vi "RunTest2.vi"(8 "error in (no error)":errorcluster, 11 "Prueba05 in":refnum<class "Prueba05.lvclass">) -> (0 "error out":errorcluster, 2 "resultado":string, 3 "Prueba05 out":refnum<class "Prueba05.lvclass">)   [LabVIEW 2019]
uses:
  Prueba/Prueba.lvclass
  Prueba05.lvclass
  <vilib>/Utility/miscctls.llb/LVRowAndColumnTypeDef.ctl
  Prueba04/Control/Slide.ctl
  Prueba04/Prueba04.lvclass
  QMH/User Event - Stop/User Event - Stop.lvlib
  QMH/Message Queue/Message Queue.lvlib
  <vilib>/Utility/error.llb/Error Cluster From Error Code.vi
  <vilib>/ErrorRing/Error Ring.xnode
  QMH/Message Queue/Enqueue Message (Single).vi
  ClusterGEN.ctl
  <vilib>/Utility/error.llb/DialogType.ctl
  D:/REPO/GitHub/procal/Pruebas/Prueba/Prueba.lvclass
panel:
  out "cumple_no_cumple":bool
  in  "Tab":enum32{"Page 1", "Page 2"}(tab)
  in  "generar_1":bool
  out "frecuencia":dbl
  in  "seguir":bool
  out "voltaje1":dbl format="%.1f"
  out "frecuencia1":dbl format="%.1f"
  in  "AjusteAmp":T1=50.0 caption="Ajuste de amplitud [mV]" scale=0.0..500.0
  in  "guardar":bool
  in  "Tabla_A":string[][](table)
  out "voltaje2":dbl format="%.1f"
  out "frecuencia2":dbl format="%.1f"
  out "no_cumple":bool
  out "cumple":bool
  out "voltaje2":dbl format="%.1f"
  in  "generar_2":bool
  out "frecuencia2":dbl
  in  "salir":bool
  # "Generación Señal de Prueba"
  # "Hz"
  # "Frecuencia"
  # "5. Ponderaciones frecuenciales y temporales a 1 KHz. IEC 61672-3: 2006 Cláusula 13"
  # "Monitoreo"
  # "Frecuencia"
  # "Hz"
  # "Voltaje"
  # "mV"
  # "Hz"
  # "mV"
  # "Cumple"
  # "No Cumple"
  # "Monitoreo"
  # "Frecuencia"
  # "Hz"
  # "Voltaje"
  # "mV"
  # "Voltaje"
  # "Frecuencia"
  # "5. Ponderaciones frecuenciales y temporales a 1 KHz. IEC 61672-3: 2006 Cláusula 13"
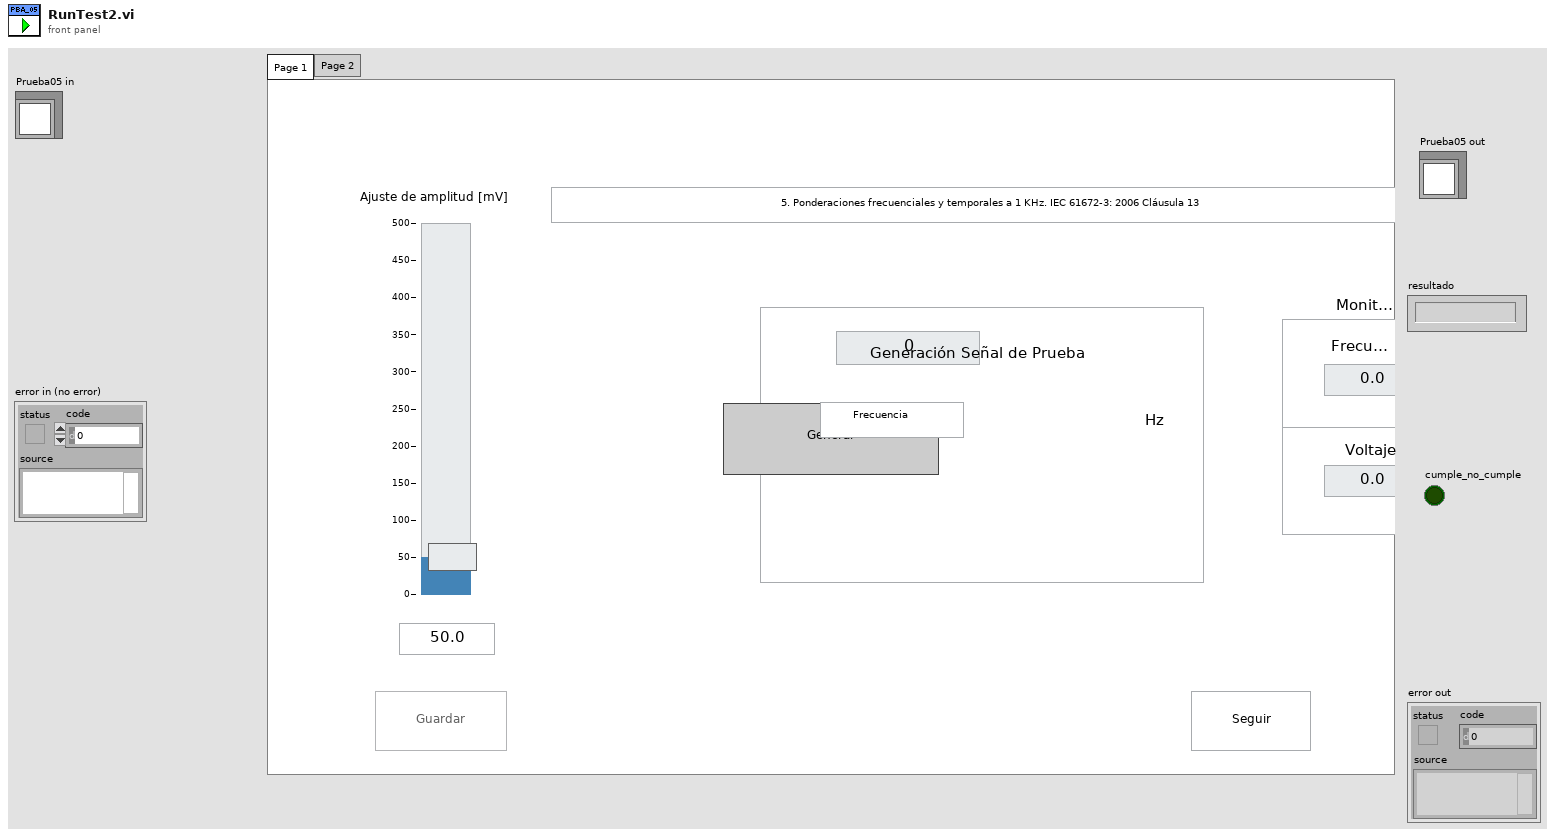
[diagram p1: front panel]
types:
  T1 = typedef "Prueba04.lvclass/Slide.ctl" = dbl
  T2 = typedef "Message Queue.lvlib/All Message Queues.ctl" = cluster{"MHL":refnum<queue>, "Inst_CNT90":refnum<queue>, "Inst_DS360":refnum<queue>, "Inst_Keithley2002":refnum<queue>, "Inst_DAQ":refnum<queue>, "BD":refnum<queue>, "Pistofono":refnum<queue>, "Nexus":refnum<queue>}
  T3 = enum8{"Enabled", "Disabled", "Disabled and Grayed Out"}
  T4 = typedef "LVRowAndColumnTypeDef.ctl" = cluster{"Row":i32, "Column":i32}
  T5 = enum32{"Page 1", "Page 2", "Page 3", "Page 4", "Page 5", "Page 6", "Page 7"}
  T6 = typedef "Prueba05.lvclass/ClusterGEN.ctl" = cluster{"frec":dbl, "amp":dbl}
  T7 = cluster{"ControlName":string, "ControlReference":refnum<vi>}[]
  T8 = typedef "DialogType.ctl" = u16
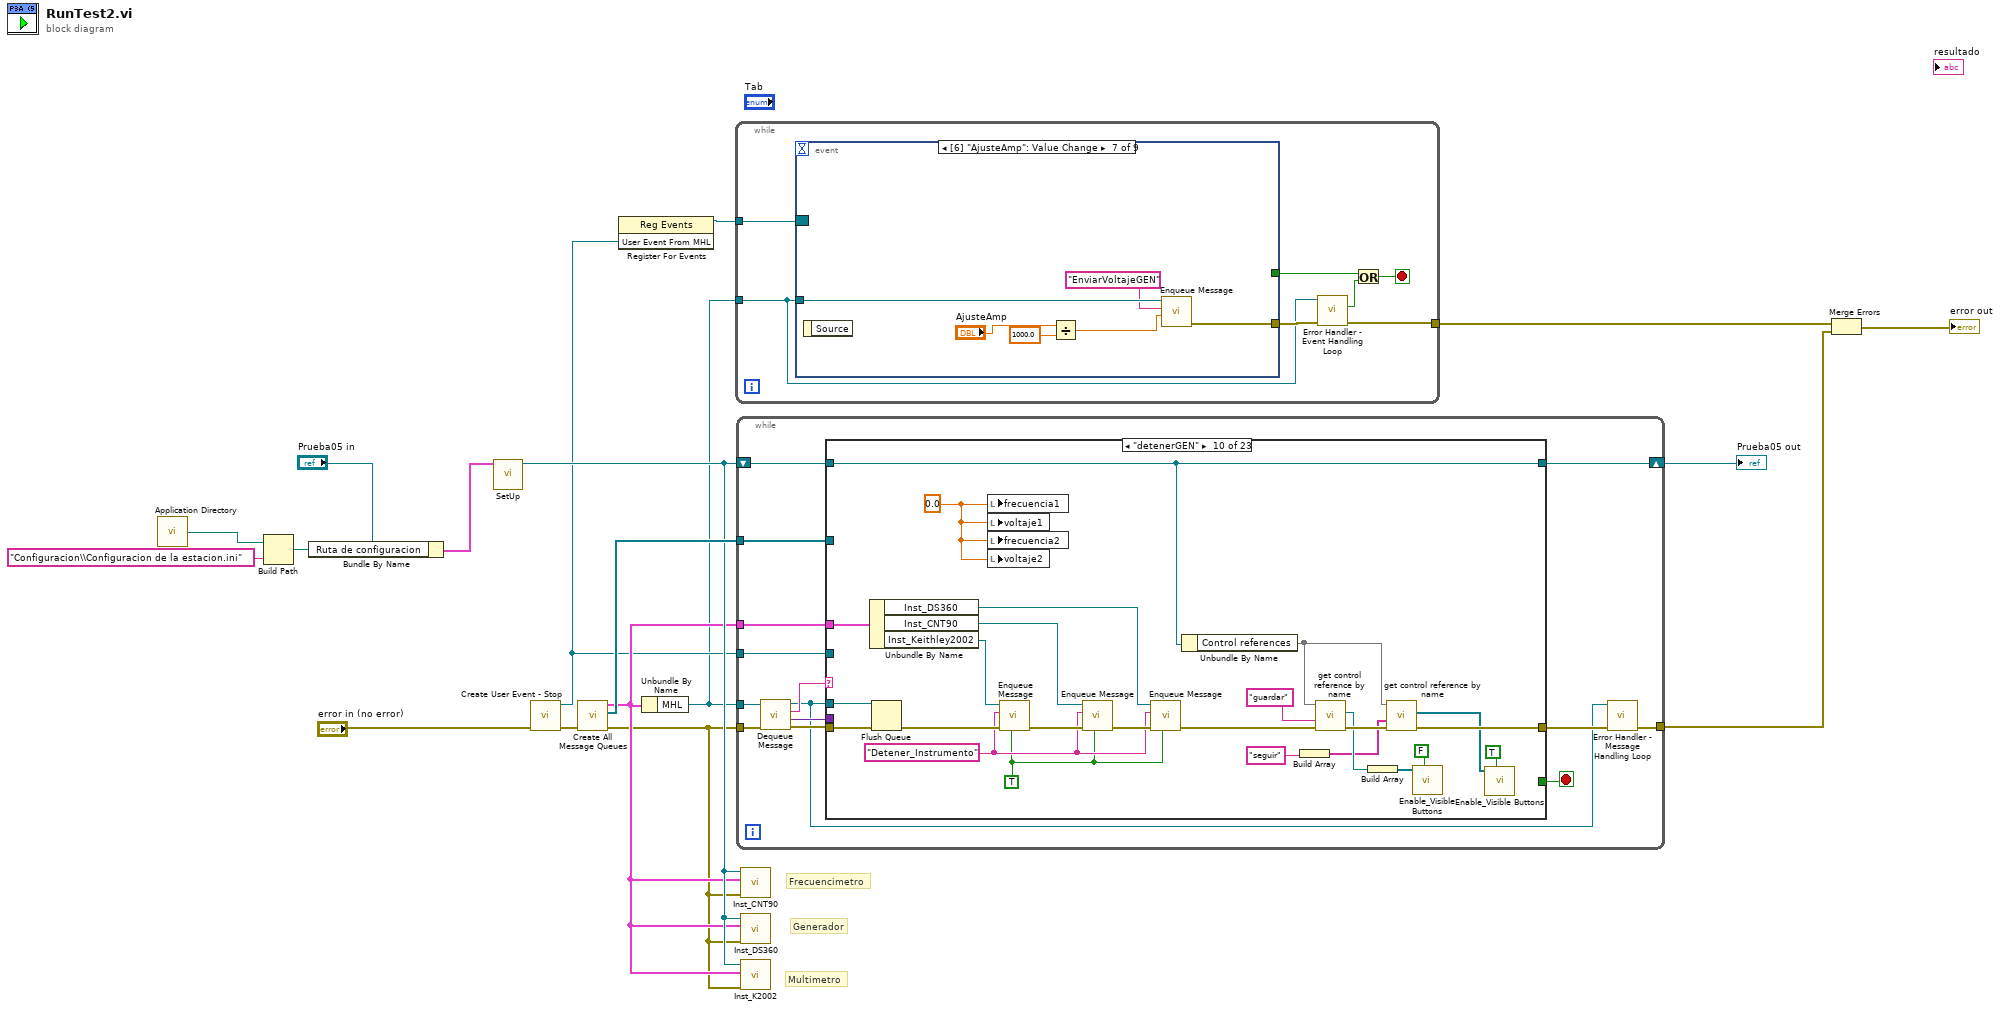
[diagram p0: block diagram]
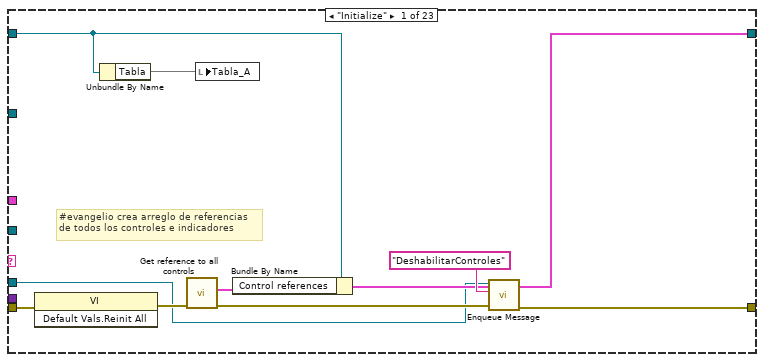
[diagram p2: hidden frame]
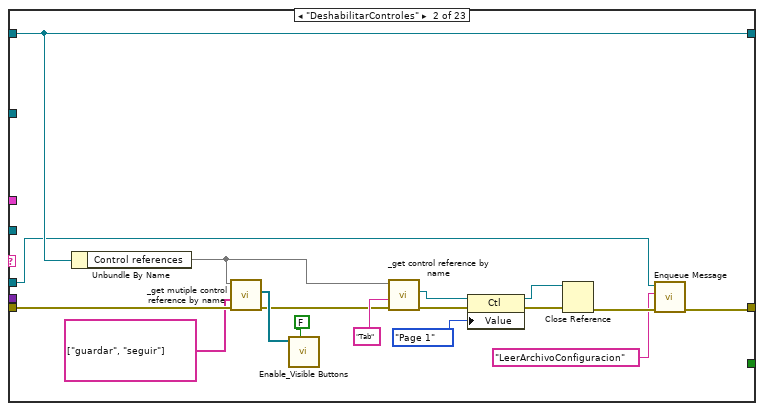
[diagram p3: hidden frame]
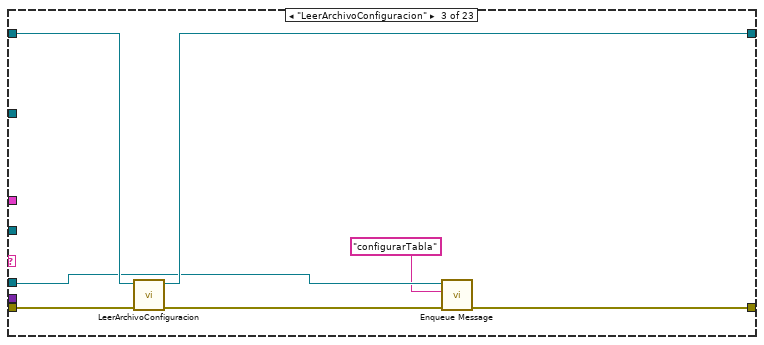
[diagram p4: hidden frame]
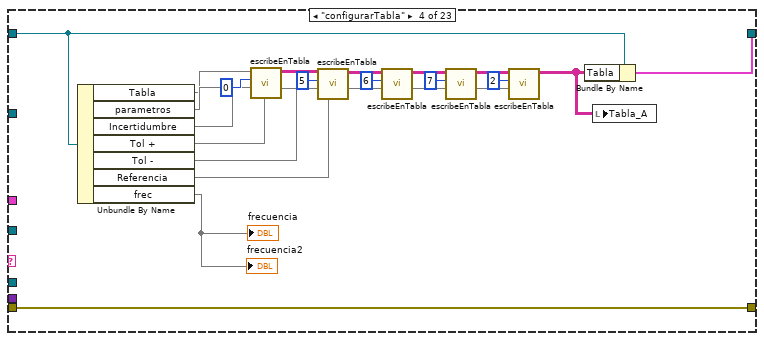
[diagram p5: hidden frame]
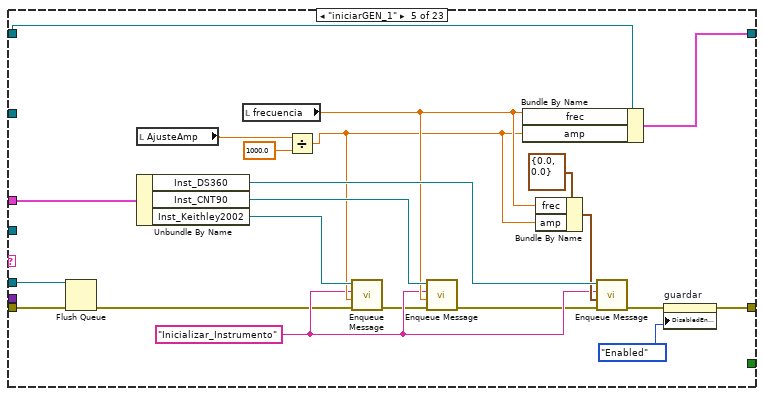
[diagram p6: hidden frame]
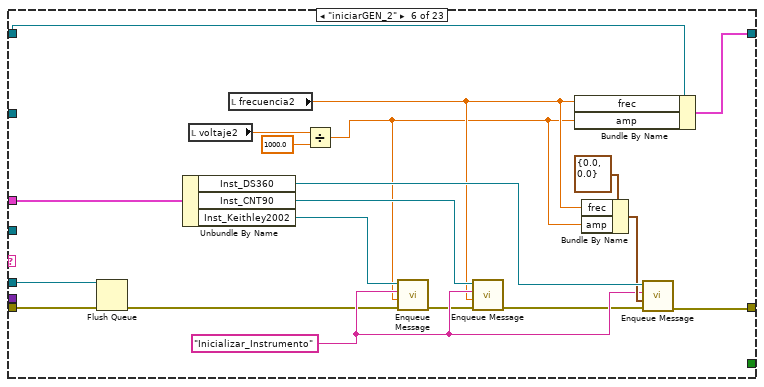
[diagram p7: hidden frame]
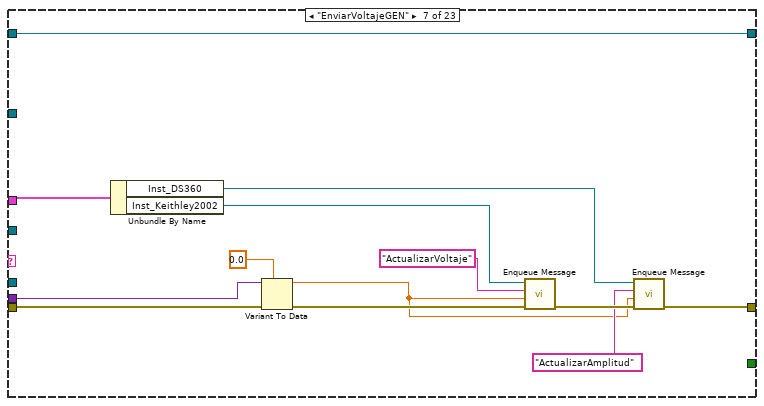
[diagram p8: hidden frame]
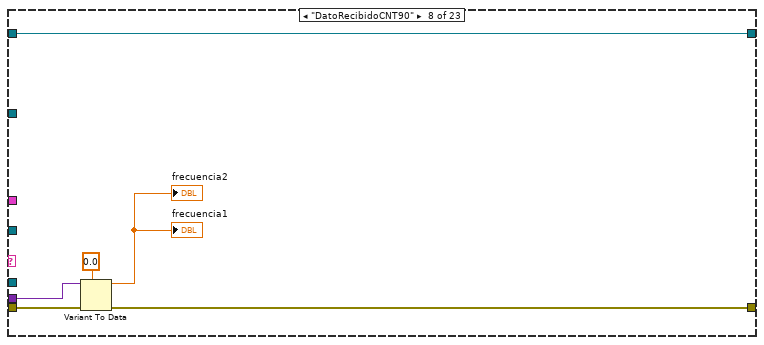
[diagram p9: hidden frame]
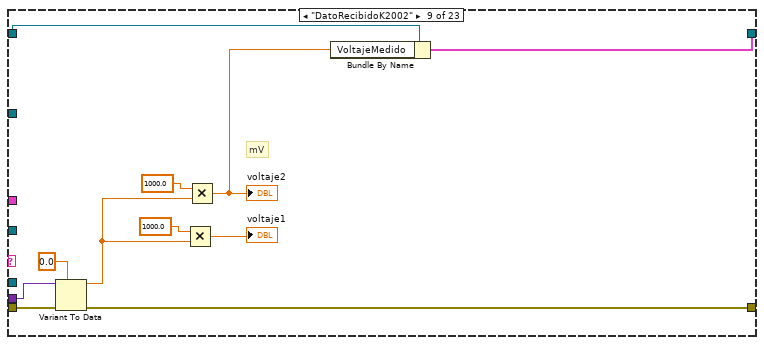
[diagram p10: hidden frame]
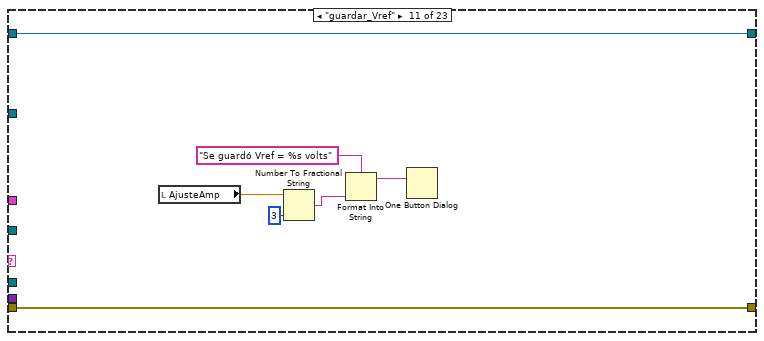
[diagram p11: hidden frame]
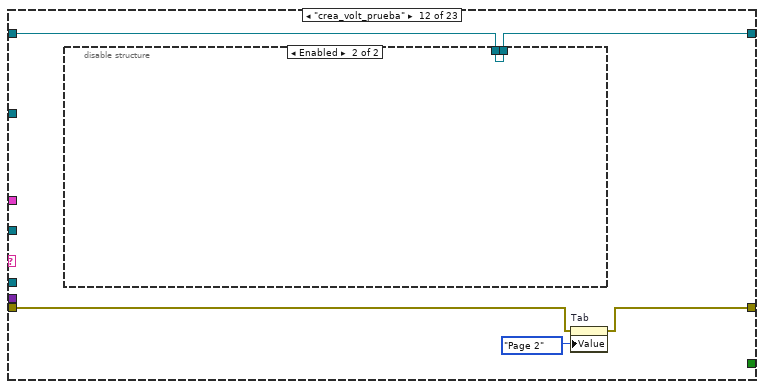
[diagram p12: hidden frame]
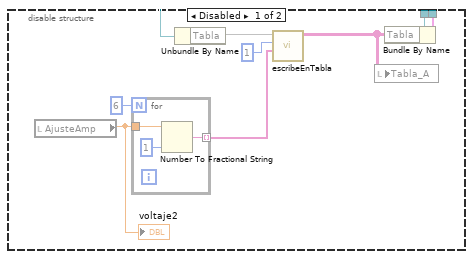
[diagram p13: hidden frame]
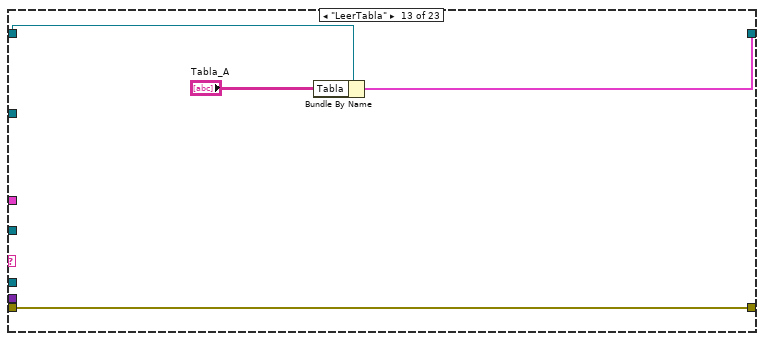
[diagram p14: hidden frame]
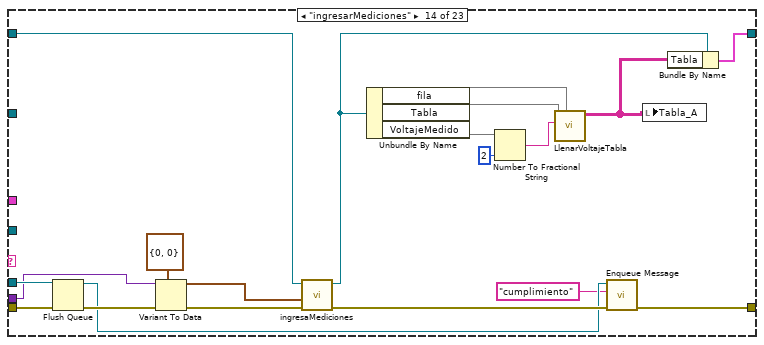
[diagram p15: hidden frame]
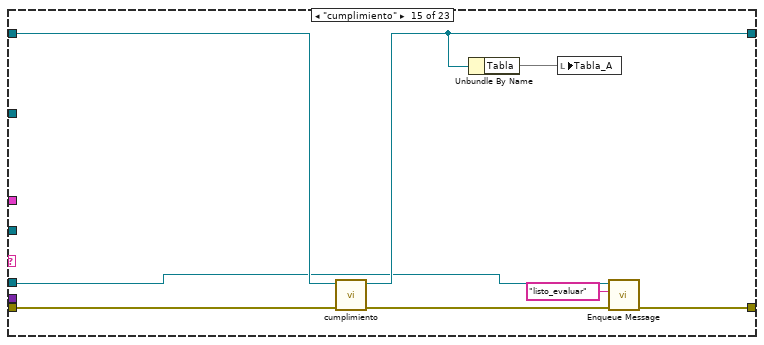
[diagram p16: hidden frame]
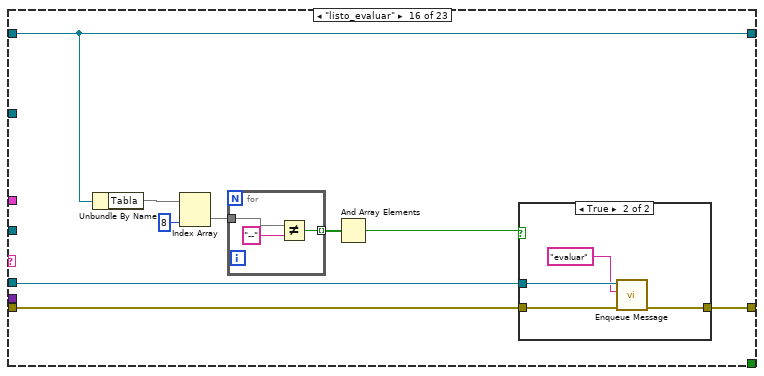
[diagram p17: hidden frame]
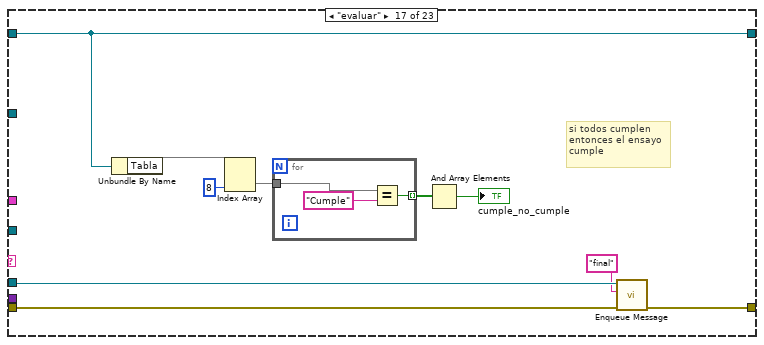
[diagram p19: hidden frame]
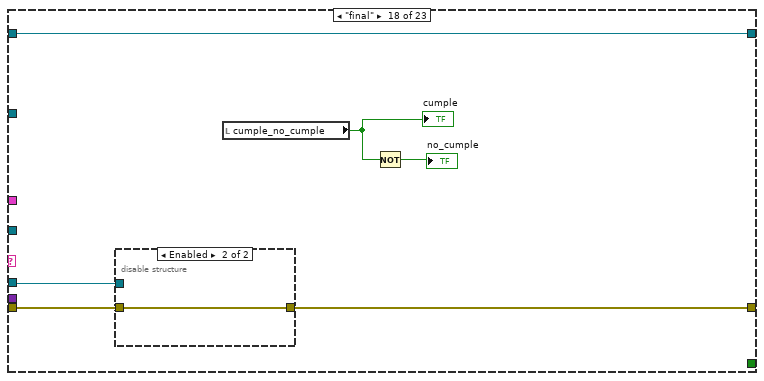
[diagram p20: hidden frame]
diagram:
  # "Multimetro"
  # "Generador"
  # "Frecuencimetro"
  n1 = call <vilib>:"Application Directory.vi"() -> ("Application Directory"=w13:path)
  n2 = Build Path(base path=w13, name or relative path="Configuracion\\Configuracion de la estacion.ini") -> (appended path=w12:path)
  n3 = Bundle By Name(cluster="Prueba05 in", "Ruta de configuracion"=w12) -> (w10:cluster{})
  n4 = call-dynamic "SetUp.vi"("Prueba05 in"=w10) -> ("Prueba05 out"=w5:refnum<class "Prueba05.lvclass">)  [unwired: 9 in, 1 out]
  n5 = call "Create User Event - Stop.vi"("error in (no error)"="error in (no error)") -> ("error out"=w9:errorcluster, "User Event From MHL"=w2:refnum<user-event>)  [unwired: 9 in]
  n6 = call "Create All Message Queues.vi"("error in (no error)"=w9) -> ("error out"=w3:errorcluster, "PL Queues Array"=w7:refnum<queue>[], "All Message Queues out"=w4:T2)  [unwired: 8 in]
  n7 = register-events(w2) -> (reference out=w6:refnum<event-registration>)  [unwired: 2 in, 1 out]
  n8 = Unbundle By Name(w4) -> ("MHL"=w1:refnum<queue>)
  n9 = while {
    tunnel: [w22] -> w18
    tunnel: w6 -> [w24]
    tunnel: w1 -> [w19]
    stop <- w25 stop-if-true
    n10 = event shown="[6] \"AjusteAmp\": Value Change" {
      selector: w24 -> [_ _ _ _ _ _ _ _ _]
      dyn-events: _ -> [_ _ _ _ _ _ _ _ _]
      timeout: _ -> [_ _ _ _ _ _ _ _ _]
      tunnel: [w28 _ w35 w39 w50 w52 w61 w62 w73] -> w23
      tunnel: w19 -> [w27 _ w37 w44 w49 w54 w60 w66 w77]
      tunnel: [_ w29 _ _ _ _ _ _ _] -> w20
      event "salir": Value Change {
        n11 = event-data() -> ()  [unwired: 1 in, 1 out]
        n12 = call-poly "Enqueue Message.vi"("Message"="Exit", "Message Queue"=w27) -> ("error out"=w28:errorcluster)  [unwired: 8 in, 1 out]
      }
      event User Event {
        n13 = event-data() -> ("User Event"=w31:string, "Event Data"=w30:variant)  [unwired: 1 in]
        n14 = case shown="\"Exit EHL\"" w31 {
          tunnel: w30 -> [_ w33]
          tunnel: [_ w32] -> w29
          frame Default {
          }
          frame "Exit EHL" {
            # "#evangelio Termina\nla ejecucion del EHL"
            n15 = Variant To Data(type=TRUE, Variant=w33) -> (data=w32:bool)  [unwired: 1 in, 1 out]
          }
        }
      }
      event Panel Close? {
        w36 = TRUE
        n16 = event-data() -> ()  [unwired: 1 in, 1 out]
        n17 = call-poly "Enqueue Message.vi"("Priority Message? (F)"=w36, "Message"="Confirmar Salida", "Message Queue"=w37) -> ("error out"=w35:errorcluster)  [unwired: 7 in, 1 out]
        n18 = event-data("Discard?"=w36) -> ()  [unwired: 1 in, 1 out]
      }
      event "generar_1": Value Change {
        n19 = event-data() -> ("NewVal"=w43:bool)  [unwired: 1 in]
        n20 = Select(t="iniciarGEN_1" ("Message"), s=w43, f="detenerGEN" ("Message")) -> (s? t:f=w40:string)
        n21 = call-poly "Enqueue Message.vi"("Message"=w40, "Message Queue"=w44) -> ("error out"=w39:errorcluster)  [unwired: 8 in, 1 out]
      }
      event "generar_2": Value Change {
        n22 = event-data() -> ("NewVal"=w48:bool)  [unwired: 1 in]
        n23 = Select(t="iniciarGEN_2", s=w48, f="detenerGEN") -> (s? t:f=w45:string)
        n24 = call-poly "Enqueue Message.vi"("Message"=w45, "Message Queue"=w49) -> ("error out"=w50:errorcluster)  [unwired: 8 in, 1 out]
      }
      event "seguir": Value Change {
        n25 = event-data() -> ()  [unwired: 1 in, 1 out]
        n26 = call-poly "Enqueue Message.vi"("Message"="crea_volt_prueba", "Message Queue"=w54) -> ("error out"=w53:errorcluster)  [unwired: 8 in, 1 out]
        n27 = property on="Tab" class="TabCtl (strict)"(error in=w53, "Value"=enum32{"Page 1", "Page 2"}."Page 2" ("Tab")) -> (error out=w52:errorcluster)  [unwired: 1 in, 1 out]
      }
      event Value Change {
        n28 = event-data() -> ()  [unwired: 1 in, 1 out]
        n29 = Divide(x="AjusteAmp", y=T1 1000.0) -> (x/y=w56:T1)
        n30 = call-poly "Enqueue Message.vi"("Message Data"=w56, "Message"="EnviarVoltajeGEN", "Message Queue"=w60) -> ("error out"=w61:errorcluster)  [unwired: 7 in, 1 out]
      }
      event "guardar": Value Change {
        n31 = event-data() -> ()  [unwired: 1 in, 1 out]
        n32 = call-poly "Enqueue Message.vi"("Message"="guardar_Vref", "Message Queue"=w66) -> ("error out"=w63:errorcluster)  [unwired: 8 in, 1 out]
        n33 = property on="seguir" class="Bool"(error in=w63, "DisabledEnum"=T3."Enabled" ("Disabled")) -> (error out=w62:errorcluster)  [unwired: 1 in, 1 out]
      }
      event "Tabla_A": Value Change {
        n34 = event-data() -> ("CtlRef"=w76:refnum<vi>)  [unwired: 1 in]
        n35 = Flush Queue(queue=w77) -> (queue out=w69:refnum<queue>, error out=w67:errorcluster)  [unwired: 1 in, 1 out]
        n36 = property class="Tbl (strict)"(reference=w76, error in=w67) -> (error out=w68:errorcluster, "Selection Start"=w72:T4)  [unwired: 1 out]
        n37 = call-poly "Enqueue Message.vi"("error in (no error)"=w68, "Message"="LeerTabla", "Message Queue"=w69) -> ("error out"=w74:errorcluster, "dup Message Queue"=w75:refnum<queue>)  [unwired: 7 in]
        n38 = call-poly "Enqueue Message.vi"("error in (no error)"=w74, "Message Data"=w72, "Message"="ingresarMediciones", "Message Queue"=w75) -> ("error out"=w73:errorcluster)  [unwired: 6 in, 1 out]
      }
    }
    n39 = call "Error Handler - Event Handling Loop.vi"("error in (no error)"=w23, "Message Queue"=w19) -> ("dup error in"=w22:errorcluster, "Error?"=w21:bool)  [unwired: 7 in, 1 out]
    n40 = Or(x=w20, y=w21) -> (x .or. y?=w25:bool)
  }
  n41 = while {
    tunnel: [w82] -> w17
    shift-right: [w90] -> w15
    shift-left: w5 -> [w91]
    tunnel: w3 -> [w89]
    tunnel: w1 -> [w87]
    tunnel: w4 -> [w81]
    tunnel: w7 -> [w80]
    tunnel: w2 -> [w79]
    stop <- w78 stop-if-true
    n42 = call "Dequeue Message.vi"("error in (no error)"=w89, "Message Queue"=w87) -> ("error out"=w88:errorcluster, "Message Data"=w85:variant, "Message"=w86:string, "dup Message Queue"=w83:refnum<queue>)  [unwired: 6 in]
    n43 = case shown="\"detenerGEN\"" w86 {
      selector: w86 -> [_ _ _ _ _ _ _ _ _ _ _ _ _ _ _ _ _ _ _ w340 _ _ w380]
      tunnel: w88 -> [w96 w113 w125 w145 w166 w185 w187 w204 w215 w230 w244 w246 w265 w285 w293 w302 w320 w329 w339 w346 w358 w372 _]
      tunnel: [w101 w104 w121 w145 w146 w170 w186 w201 w211 w225 w244 w245 w265 w283 w291 w298 w315 w325 w335 w345 w356 w370 w379] -> w84
      tunnel: w83 -> [w92 w103 w120 _ w161 w180 _ _ _ w229 _ _ _ w276 w287 w295 w312 w324 w337 w347 w357 w371 _]
      tunnel: w91 -> [w95 w112 w123 w129 w165 w184 w198 w203 w214 w216 w238 w248 w264 w279 w290 w297 w314 w326 w338 w342 w363 w378 w381]
      tunnel: [w94 w112 w122 w127 w164 w183 w198 w203 w206 w216 w238 w249 w263 w266 w289 w297 w314 w326 w338 w342 w363 w378 w381] -> w90
      tunnel: w85 -> [_ _ _ _ _ _ w188 w202 w210 _ _ _ _ w274 _ _ _ _ _ _ _ w369 _]
      tunnel: w81 -> [_ _ _ _ w159 w173 w189 _ _ w228 _ _ _ _ _ _ _ _ _ _ _ _ _]
      tunnel: w80 -> [_ _ _ _ _ _ _ _ _ _ _ _ _ _ _ _ _ _ _ w343 _ _ _]
      tunnel: w79 -> [_ _ _ _ _ _ _ _ _ _ _ _ _ _ _ _ _ _ _ w344 _ _ _]
      tunnel: [_ _ _ _ _ _ _ _ _ _ _ _ _ _ _ _ _ _ _ w341 _ _ _] -> w78
      frame "Initialize" {
        # "#evangelio crea arreglo de referencias\nde todos los controles e indicadores"
        n44 = invoke class="VI" method="Default Vals.Reinit All"(error in=w96) -> (error out=w98:errorcluster)  [unwired: 2 in, 2 out]
        n45 = Unbundle By Name(w95) -> ("Tabla"=w100)
        n46 = call "Get reference to all controls.vi"("error in (no error)"=w98) -> ("error out"=w93:errorcluster, "Control references"=w97:T7)  [unwired: 5 in]
        n47 = local write "Tabla_A"(w100) -> ()
        n48 = Bundle By Name(cluster=w95, "Control references"=w97) -> (w94:cluster{})
        n49 = call-poly "Enqueue Message.vi"("error in (no error)"=w93, "Message"="DeshabilitarControles", "Message Queue"=w92) -> ("error out"=w101:errorcluster)  [unwired: 7 in, 1 out]
      }
      frame "DeshabilitarControles" {
        n50 = Unbundle By Name(w112) -> ("Control references"=w114)
        n51 = call "_get mutiple control reference by name.vi"("error in (no error)"=w113, "Control names"=string[] ["guardar", "seguir"], "Control references"=w114) -> ("error out"=w109:errorcluster, "References"=w110:refnum<vi>[])  [unwired: 3 in]
        n52 = call "Enable_Visible Buttons.vi"("Enable? (T)"=FALSE, "Controls Ref Array"=w110) -> ()  [unwired: 10 in]
        n53 = call "_get control reference by name.vi"("error in (no error)"=w109, "Control name"="Tab" ("Message"), "Control references"=w114) -> ("error out"=w118:errorcluster, "Ctl Refnum"=w116:refnum<vi>)  [unwired: 3 in]
        n54 = property class="Ctl"(reference=w116, error in=w118, "Value"=T5."Page 1" ("Tab_Prueba04")) -> (reference out=w105:refnum<vi>, error out=w107:errorcluster)
        n55 = Close Reference(reference=w105, error in (no error)=w107) -> (error out=w106:errorcluster)
        n56 = call-poly "Enqueue Message.vi"("error in (no error)"=w106, "Message"="LeerArchivoConfiguracion", "Message Queue"=w103) -> ("error out"=w104:errorcluster)  [unwired: 7 in, 1 out]
      }
      frame "LeerArchivoConfiguracion" {
        n57 = call "LeerArchivoConfiguracion.vi"("error in"=w125, "Prueba05 in"=w123) -> ("error out"=w124:errorcluster, "Prueba05 out"=w122:refnum<class "Prueba05.lvclass">)  [unwired: 8 in]
        n58 = call-poly "Enqueue Message.vi"("error in (no error)"=w124, "Message"="configurarTabla", "Message Queue"=w120) -> ("error out"=w121:errorcluster)  [unwired: 7 in, 1 out]
      }
      frame "configurarTabla" {
        n59 = Unbundle By Name(w129) -> ("Tabla"=w128, "parametros"=w143, "Incertidumbre"=w136, "Tol +"=w135, "Tol -"=w134, "Referencia"=w131, "frec"=→"frecuencia" →"frecuencia2")
        n60 = call "escribeEnTabla.vi"("parametros"=w143, "col"=0, "tabla in"=w128) -> ("tabla out"=w137:string[][])  [unwired: 8 in]
        n61 = call "escribeEnTabla.vi"("parametros"=w136, "col"=5, "tabla in"=w137) -> ("tabla out"=w142:string[][])  [unwired: 8 in]
        n62 = call "escribeEnTabla.vi"("parametros"=w135, "col"=6, "tabla in"=w142) -> ("tabla out"=w141:string[][])  [unwired: 8 in]
        n63 = call "escribeEnTabla.vi"("parametros"=w134, "col"=7, "tabla in"=w141) -> ("tabla out"=w132:string[][])  [unwired: 8 in]
        n64 = call "escribeEnTabla.vi"("parametros"=w131, "col"=2, "tabla in"=w132) -> ("tabla out"=w126:string[][])  [unwired: 8 in]
        n65 = Bundle By Name(cluster=w129, "Tabla"=w126) -> (w127:cluster{})
        n66 = local write "Tabla_A"(w126) -> ()
      }
      frame "iniciarGEN_1" {
        w152 = "Inicializar_Instrumento" ("Message")
        n67 = Flush Queue(queue=w161, error in (no error)=w166) -> (error out=w151:errorcluster)  [unwired: 2 out]
        n68 = local read "AjusteAmp"() -> (w162:T1)
        n69 = Unbundle By Name(w159) -> ("Inst_DS360"=w158:refnum<queue>, "Inst_CNT90"=w157:refnum<queue>, "Inst_Keithley2002"=w156:refnum<queue>)
        n70 = local read "frecuencia"() -> (w154:dbl)
        n71 = Divide(x=w162, y=T1 1000.0) -> (x/y=w153:T1)
        n72 = call-poly "Enqueue Message.vi"("error in (no error)"=w151, "Message Data"=w153, "Message"=w152, "Message Queue"=w156) -> ("error out"=w150:errorcluster)  [unwired: 6 in, 1 out]
        n73 = call-poly "Enqueue Message.vi"("error in (no error)"=w150, "Message Data"=w154, "Message"=w152, "Message Queue"=w157) -> ("error out"=w149:errorcluster)  [unwired: 6 in, 1 out]
        n74 = Bundle By Name(cluster=w165, "frec"=w154, "amp"=w153) -> (w164:cluster{})
        n75 = Bundle By Name(cluster=T6 {"frec"=0.0, "amp"=0.0}, "frec"=w154, "amp"=w153) -> (w155:T6)
        n76 = call-poly "Enqueue Message.vi"("error in (no error)"=w149, "Message Data"=w155, "Message"=w152, "Message Queue"=w158) -> ("error out"=w147:errorcluster)  [unwired: 6 in, 1 out]
        n77 = property on="guardar" class="Bool"(error in=w147, "DisabledEnum"=T3."Enabled" ("Disabled")) -> (error out=w146:errorcluster)  [unwired: 1 in, 1 out]
      }
      frame "iniciarGEN_2" {
        w174 = "Inicializar_Instrumento" ("Message")
        n78 = Flush Queue(queue=w180, error in (no error)=w185) -> (error out=w169:errorcluster)  [unwired: 2 out]
        n79 = Unbundle By Name(w173) -> ("Inst_DS360"=w178:refnum<queue>, "Inst_CNT90"=w177:refnum<queue>, "Inst_Keithley2002"=w176:refnum<queue>)
        n80 = local read "voltaje2"() -> (w181:dbl)
        n81 = local read "frecuencia2"() -> (w172:dbl)
        n82 = Divide(x=w181, y=T1 1000.0) -> (x/y=w171:T1)
        n83 = call-poly "Enqueue Message.vi"("error in (no error)"=w169, "Message Data"=w171, "Message"=w174, "Message Queue"=w176) -> ("error out"=w168:errorcluster)  [unwired: 6 in, 1 out]
        n84 = call-poly "Enqueue Message.vi"("error in (no error)"=w168, "Message Data"=w172, "Message"=w174, "Message Queue"=w177) -> ("error out"=w167:errorcluster)  [unwired: 6 in, 1 out]
        n85 = Bundle By Name(cluster=w184, "frec"=w172, "amp"=w171) -> (w183:cluster{})
        n86 = Bundle By Name(cluster=T6 {"frec"=0.0, "amp"=0.0}, "frec"=w172, "amp"=w171) -> (w175:T6)
        n87 = call-poly "Enqueue Message.vi"("error in (no error)"=w167, "Message Data"=w175, "Message"=w174, "Message Queue"=w178) -> ("error out"=w170:errorcluster)  [unwired: 6 in, 1 out]
      }
      frame "EnviarVoltajeGEN" {
        n88 = Unbundle By Name(w189) -> ("Inst_DS360"=w192:refnum<queue>, "Inst_Keithley2002"=w197:refnum<queue>)
        n89 = Variant To Data(error in=w187, type=0.0, Variant=w188) -> (data=w190:dbl, error out=w195:errorcluster)
        n90 = call-poly "Enqueue Message.vi"("error in (no error)"=w195, "Message Data"=w190, "Message"="ActualizarVoltaje", "Message Queue"=w197) -> ("error out"=w193:errorcluster)  [unwired: 6 in, 1 out]
        n91 = call-poly "Enqueue Message.vi"("error in (no error)"=w193, "Message Data"=w190, "Message"="ActualizarAmplitud", "Message Queue"=w192) -> ("error out"=w186:errorcluster)  [unwired: 6 in, 1 out]
      }
      frame "DatoRecibidoCNT90" {
        n92 = Variant To Data(error in=w204, type=0.0, Variant=w202) -> (data=→"frecuencia2" →"frecuencia1":dbl, error out=w201:errorcluster)
      }
      frame "DatoRecibidoK2002" {
        # "mV"
        n93 = Variant To Data(error in=w215, type=0.0 ("x"), Variant=w210) -> (data=w207:dbl, error out=w211:errorcluster)
        n94 = Multiply(x=1000.0, y=w207) -> (x*y=→"voltaje1":dbl)
        n95 = Multiply(x=1000.0, y=w207) -> (x*y=w205:dbl)
        "voltaje2" <- w205
        n96 = Bundle By Name(cluster=w214, "VoltajeMedido"=w205) -> (w206:cluster{})
      }
      frame "detenerGEN" {
        w231 = TRUE ("Priority Message? (F)")
        w232 = "Detener_Instrumento"
        w237 = 0.0 ("frecuencia1")
        n97 = Unbundle By Name(w228) -> ("Inst_DS360"=w233:refnum<queue>, "Inst_CNT90"=w234:refnum<queue>, "Inst_Keithley2002"=w235:refnum<queue>)
        n98 = Flush Queue(queue=w229, error in (no error)=w230) -> (error out=w236:errorcluster)  [unwired: 2 out]
        n99 = local write "frecuencia1"(w237) -> ()
        n100 = local write "voltaje1"(w237) -> ()
        n101 = local write "frecuencia2"(w237) -> ()
        n102 = local write "voltaje2"(w237) -> ()
        n103 = call-poly "Enqueue Message.vi"("Priority Message? (F)"=w231, "Message"=w232, "Message Queue"=w235) -> ()  [unwired: 7 in, 2 out]
        n104 = call-poly "Enqueue Message.vi"("Priority Message? (F)"=w231, "Message"=w232, "Message Queue"=w234) -> ()  [unwired: 7 in, 2 out]
        n105 = call-poly "Enqueue Message.vi"("Priority Message? (F)"=w231, "error in (no error)"=w236, "Message"=w232, "Message Queue"=w233) -> ("error out"=w226:errorcluster)  [unwired: 6 in, 1 out]
        n106 = Unbundle By Name(w216) -> ("Control references"=w220)
        n107 = Build Array("seguir" ("String")) -> (w217:string[])
        n108 = call-poly "get control reference by name.vi"("error in (no error)"=w226, "Control name"="guardar" ("String"), "Control references"=w220) -> ("error out"=w225:errorcluster, "Ctl Refnum"=w223:refnum<vi>)  [unwired: 3 in]
        n109 = Build Array(w223) -> (w222:refnum<vi>[])
        n110 = call-poly "get control reference by name.vi"("Control names"=w217, "Control references"=w220) -> ("References"=w219:refnum<vi>[])  [unwired: 4 in, 1 out]
        n111 = call "Enable_Visible Buttons.vi"("Enable? (T)"=FALSE, "Controls Ref Array"=w222) -> ()  [unwired: 10 in]
        n112 = call "Enable_Visible Buttons.vi"("Enable? (T)"=TRUE, "Controls Ref Array"=w219) -> ()  [unwired: 10 in]
      }
      frame "guardar_Vref" {
        n113 = local read "AjusteAmp"() -> (w239:T1)
        n114 = Number To Fractional String(number=w239, precision (6)=i16 3) -> (F-format string=w240:string)  [unwired: 2 in]
        n115 = Format Into String(format string="Se guardó Vref = %s volts", w240) -> (resulting string=w243:string)  [unwired: 2 in, 1 out]
        n116 = One Button Dialog(message=w243) -> ()  [unwired: 1 in, 1 out]
      }
      frame "crea_volt_prueba" {
        n117 = disable-structure shown="Enabled" {
          disable-tunnel: [w253 w261] -> w249
          disable-tunnel: w248 -> [w252 w261]
          frame Disabled {
            n118 = local read "AjusteAmp"() -> (w254:T1)
            "voltaje2" <- w254
            n119 = for {
              N: 6 -> [_]
              tunnel: w254 -> [w260]
              tunnel: [w258] -> w255 mode=indexing
              n120 = Number To Fractional String(number=w260, precision (6)=i16 1) -> (F-format string=w258:string)  [unwired: 2 in]
            }
            n121 = Unbundle By Name(w252) -> ("Tabla"=w251)
            n122 = call "escribeEnTabla.vi"("parametros"=w255, "col"=1, "tabla in"=w251) -> ("tabla out"=w250:string[][])  [unwired: 8 in]
            n123 = local write "Tabla_A"(w250) -> ()
            n124 = Bundle By Name(cluster=w252, "Tabla"=w250) -> (w253:cluster{})
          }
          frame Enabled {
          }
        }
        n125 = property on="Tab" class="TabCtl (strict)"(error in=w246, "Value"=enum32{"Page 1", "Page 2"}."Page 2" ("Tab")) -> (error out=w245:errorcluster)  [unwired: 1 in, 1 out]
      }
      frame "LeerTabla" {
        n126 = Bundle By Name(cluster=w264, "Tabla"="Tabla_A") -> (w263:cluster{})
      }
      frame "ingresarMediciones" {
        n127 = Flush Queue(queue=w276, error in (no error)=w285) -> (queue out=w280:refnum<queue>, error out=w281:errorcluster)  [unwired: 1 out]
        n128 = Variant To Data(error in=w281, type=T4 {"Row"=0, "Column"=0} ("Selection Start"), Variant=w274) -> (data=w277:T4, error out=w282:errorcluster)
        n129 = call "ingresaMediciones.vi"("error in (no error)"=w282, "Selection Start"=w277, "Prueba05 in"=w279) -> ("error out"=w284:errorcluster, "Prueba05 out"=w267:refnum<class "Prueba05.lvclass">)  [unwired: 7 in]
        n130 = Unbundle By Name(w267) -> ("fila"=w269, "Tabla"=w272, "VoltajeMedido"=w273)
        n131 = Number To Fractional String(number=w273, precision (6)=i16 2) -> (F-format string=w271:string)  [unwired: 2 in]
        n132 = call "LlenarVoltajeTabla.vi"("fila"=w269, "Dato"=w271, "Tabla in"=w272) -> ("Tabla out"=w270:string[][])  [unwired: 8 in]
        n133 = call-poly "Enqueue Message.vi"("error in (no error)"=w284, "Message"="cumplimiento", "Message Queue"=w280) -> ("error out"=w283:errorcluster)  [unwired: 7 in, 1 out]
        n134 = local write "Tabla_A"(w270) -> ()
        n135 = Bundle By Name(cluster=w267, "Tabla"=w270) -> (w266:cluster{})
      }
      frame "cumplimiento" {
        n136 = call "cumplimiento.vi"("error in (no error)"=w293, "Prueba04 in"=w290) -> ("error out"=w292:errorcluster, "Prueba04 out"=w289:refnum<class "Prueba05.lvclass">)  [unwired: 8 in]
        n137 = Unbundle By Name(w289) -> ("Tabla"=w288)
        n138 = local write "Tabla_A"(w288) -> ()
        n139 = call-poly "Enqueue Message.vi"("error in (no error)"=w292, "Message"="listo_evaluar", "Message Queue"=w287) -> ("error out"=w291:errorcluster)  [unwired: 7 in, 1 out]
      }
      frame "listo_evaluar" {
        n140 = Unbundle By Name(w297) -> ("Tabla"=w296)
        n141 = Index Array(array=w296, index (col)=8 ("disabled index (col)")) -> (element=w300)  [unwired: 1 in]
        n142 = for {
          tunnel: [w310] -> w299 mode=indexing
          tunnel: w300 -> [w308]
          n143 = Not Equal?(x=w308, y="--") -> (x != y?=w310:bool)
        }
        n144 = And Array Elements(Boolean array=w299) -> (logical AND=w294:bool)
        n145 = case shown="True" w294 {
          tunnel: w302 -> [w303 w307]
          tunnel: [w303 w306] -> w298
          tunnel: w295 -> [_ w305]
          frame False {
          }
          frame True {
            n146 = call-poly "Enqueue Message.vi"("error in (no error)"=w307, "Message"="evaluar", "Message Queue"=w305) -> ("error out"=w306:errorcluster)  [unwired: 7 in, 1 out]
          }
        }
      }
      frame "evaluar" {
        # "si todos cumplen\nentonces el ensayo\ncumple"
        n147 = Unbundle By Name(w314) -> ("Tabla"=w313)
        n148 = Index Array(array=w313, index (col)=8 ("disabled index (col)")) -> (element=w317)  [unwired: 1 in]
        n149 = for {
          tunnel: [w323] -> w318 mode=indexing
          tunnel: w317 -> [w321]
          n150 = Equal?(x=w321, y="Cumple") -> (x = y?=w323:bool)
        }
        n151 = And Array Elements(Boolean array=w318) -> (logical AND=→"cumple_no_cumple":bool)
        n152 = call-poly "Enqueue Message.vi"("error in (no error)"=w320, "Message"="final", "Message Queue"=w312) -> ("error out"=w315:errorcluster)  [unwired: 7 in, 1 out]
      }
      frame "final" {
        n153 = disable-structure shown="Enabled" {
          disable-tunnel: w329 -> [w333 w334]
          disable-tunnel: [w332 w334] -> w325
          disable-tunnel: w324 -> [w331 _]
          frame Disabled {
            n154 = call-poly "Enqueue Message.vi"("error in (no error)"=w333, "Message"="detenerGEN", "Message Queue"=w331) -> ("error out"=w332:errorcluster)  [unwired: 7 in, 1 out]
          }
          frame Enabled {
          }
        }
        n155 = local read "cumple_no_cumple"() -> (w327:bool)
        "cumple" <- w327
        n156 = Not(x=w327) -> (.not. x?=→"no_cumple":bool)
      }
      frame "DetieneInstrumentos" {
        n157 = call-poly "Enqueue Message.vi"("error in (no error)"=w339, "Message"="salir", "Message Queue"=w337) -> ("error out"=w335:errorcluster)  [unwired: 7 in, 1 out]
      }
      frame "Exit" {
        w341 = TRUE
        # "#evangelio Manda a cerrar el EHL"
        # "#evangelio Manda a cerrar todos los Loops"
        n158 = Release Queue(queue=w347, error in (no error)=w346) -> (error out=w351:errorcluster)  [unwired: 1 in, 2 out]
        n159 = Unbundle By Name(w342) -> ("Control references"=w352)
        n160 = for {
          tunnel: w343 -> [w355] mode=indexing
          tunnel: w340 -> [w354]
          tunnel: TRUE -> [w353]
          n161 = call-poly "Enqueue Message.vi"("Priority Message? (F)"=w353, "Message"=w354, "Message Queue"=w355) -> ()  [unwired: 7 in, 2 out]
        }
        n162 = call "Close All Ref.vi"("error in (no error)"=w351, "Control references"=w352) -> ("error out"=w349:errorcluster)  [unwired: 9 in]
        n163 = call "Fire User Event - Stop.vi"("error in (no error)"=w349, "Event Data"=w341, "User Event"="Exit EHL", "User Event in"=w344) -> ("error out"=w345:errorcluster)  [unwired: 7 in]
      }
      frame "Confirmar Salida" {
        n164 = Two Button Dialog(message="¿Quieres cerrar la aplicación?", 1:"No" ("T button name (\"OK\")"), 2:"Si" ("T button name (\"OK\")")) -> (T button?=w359:bool)
        n165 = case shown="True" w359 {
          tunnel: w358 -> [w364 w368]
          tunnel: [w364 w367] -> w356
          tunnel: w357 -> [_ w365]
          frame False {
          }
          frame True {
            n166 = call-poly "Enqueue Message.vi"("error in (no error)"=w368, "Message"="Exit", "Message Queue"=w365) -> ("error out"=w367:errorcluster)  [unwired: 7 in, 1 out]
          }
        }
      }
      frame "Error" {
        w376 = T8 1 items=["no dialog", "OK message", "continue or stop message", "OK message + warnings", "continue/stop + warnings"] ("type of dialog (OK msg:1)")
        n167 = Variant To Data(error in=w372, type=errorcluster {"status"=FALSE, "code"=0, "source"=""} ("error out"), Variant=w369) -> (data=w374:errorcluster, error out=w373:errorcluster)
        n168 = call <vilib>:"Simple Error Handler.vi"("type of dialog (OK msg:1)"=w376, "error in (no error)"=w374) -> ()  [unwired: 3 in, 5 out]
        n169 = call-poly "Enqueue Message.vi"("error in (no error)"=w373, "Message"="Exit", "Message Queue"=w371) -> ("error out"=w370:errorcluster)  [unwired: 7 in, 1 out]
      }
      frame Default {
        n170 = xnode "Error Ring"("parameter 0"=w380) -> ("error out"=w379:errorcluster)
      }
    }
    n171 = call "Error Handler - Message Handling Loop.vi"("error in (no error)"=w84, "Message Queue"=w83) -> ("dup error in"=w82:errorcluster)  [unwired: 8 in, 1 out]
  }
  "Prueba05 out" <- w15
  n172 = call "Inst_CNT90.vi"("error in"=w3, "All Message Queues in"=w4, "Prueba31 in"=w5) -> ()  [unwired: 8 in, 1 out]
  n173 = call "Inst_DS360.vi"("error in"=w3, "All Message Queues in"=w4, "Prueba05 in"=w5) -> ()  [unwired: 8 in, 1 out]
  n174 = call "Inst_K2002.vi"("error in"=w3, "All Message Queues in"=w4, "Prueba31 in"=w5) -> ()  [unwired: 8 in, 1 out]
  n175 = Merge Errors(w18, w17) -> (→"error out":errorcluster)
